vi "Initialize.vi"(8 "error in (no error)":errorcluster, 10 "CommandText":string, 11 "PathCommands.LineTo in":refnum<class "PathCommands.LineTo.lvclass">) -> (0 "error out":errorcluster, 3 "PathCommands.LineTo out":refnum<class "PathCommands.LineTo.lvclass">)   [LabVIEW 2019, in "PathCommands.LineTo.lvclass"]
uses:
  PathCommands.LineTo.lvclass
  PathCommands/PathCommands.lvclass
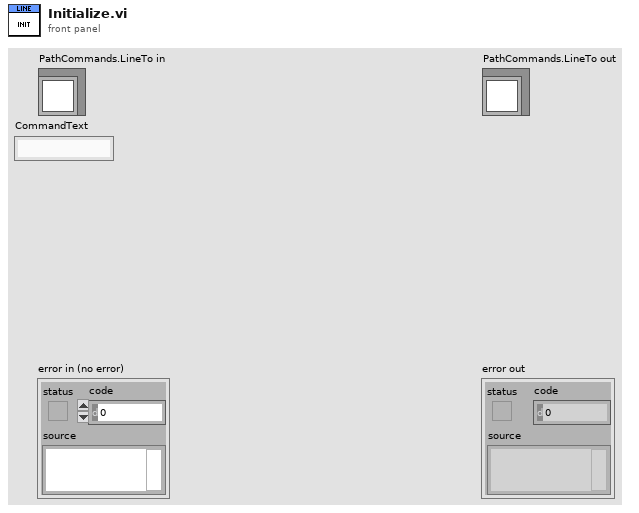
[diagram p1: front panel]
types:
  T1 = enum16{"None", "After", "Before", "Last", "First"}[]
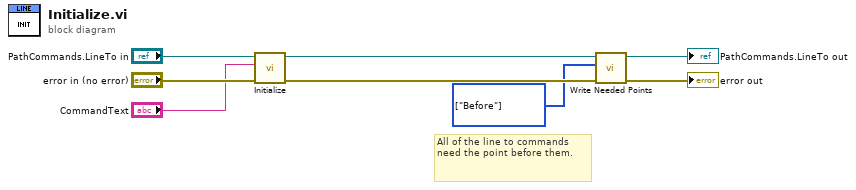
[diagram p0: block diagram]
diagram:
  w2 = T1 [enum."Before"] items=["None", "After", "Before", "Last", "First"] ("Needed Points")
  # "All of the line to commands need the point before them."
  n1 = call-parent "Initialize.vi"("error in (no error)"="error in (no error)", "CommandText"="CommandText", "PathCommands in"="PathCommands.LineTo in") -> ("error out"=w6:errorcluster, "PathCommands out"=w1:refnum<class "PathCommands.LineTo.lvclass">)  [unwired: 7 in]
  n2 = call-dynamic "Write Needed Points.vi"("error in (no error)"=w6, "Needed Points"=w2, "PathCommands in"=w1) -> ("error out"=→"error out":errorcluster, "PathCommands out"=→"PathCommands.LineTo out":refnum<class "PathCommands.LineTo.lvclass">)  [unwired: 7 in]
